vi "Get Property Node Reference.vi"(8 "error in (no error)":errorcluster) -> (0 "error out":errorcluster, 2 "Secondary Prop Refnum":refnum<vi>, 3 "Main Prop Refnum":refnum<vi>)   [LabVIEW 2023]
doc: "<b> </b> <b> </b>\n© 2017 Q Software Innovations, LLC\nwritten by Quentin \"Q\" Alldredge\nproduced in LabVIEW 2015\n\nsupport@qsoftwareinnovations.com\nwww.qsoftwareinnovations.com\n\nAll rights reserved.\n\nRedistribution and use in source and binary forms, with or without modification, are permitted provided that the following conditions are met:\n\n * Redistributions of source code must retain the above copyright notice, this list of conditions and the following disclaimer.\n * Redistributions in binary form must reproduce the above copyright notice, this list of conditions and the following disclaimer in the documentation and/or other materials provided with the distribution.\n * Neither the name of Q Software Innovations, LLC. nor the names of its contributors may be used to endorse or promote products derived from this software without specific prior written permission.\n\nTHIS SOFTWARE IS PROVIDED BY THE COPYRIGHT HOLDERS AND CONTRIBUTORS \"AS IS\" AND ANY EXPRESS OR IMPLIED WARRANTIES, INCLUDING, BUT NOT LIMITED TO, THE IMPLIED WARRANTIES OF MERCHANTABILITY AND FITNESS FOR A PARTICULAR PURPOSE ARE DISCLAIMED. IN NO EVENT SHALL THE COPYRIGHT OWNER OR CONTRIBUTORS BE LIABLE FOR ANY DIRECT, INDIRECT, INCIDENTAL, SPECIAL, EXEMPLARY, OR CONSEQUENTIAL DAMAGES (INCLUDING, BUT NOT LIMITED TO, PROCUREMENT OF SUBSTITUTE GOODS OR SERVICES; LOSS OF USE, DATA, OR PROFITS; OR BUSINESS INTERRUPTION) HOWEVER CAUSED AND ON ANY THEORY OF LIABILITY, WHETHER IN CONTRACT, STRICT LIABILITY, OR TORT (INCLUDING NEGLIGENCE OR OTHERWISE) ARISING IN ANY WAY OUT OF THE USE OF THIS SOFTWARE, EVEN IF ADVISED OF THE POSSIBILITY OF SUCH DAMAGE."
uses:
  <vilib>/Utility/traverseref.llb/VI Scripting - Traverse.lvlib
panel:
  out "exe time (ms)":u32
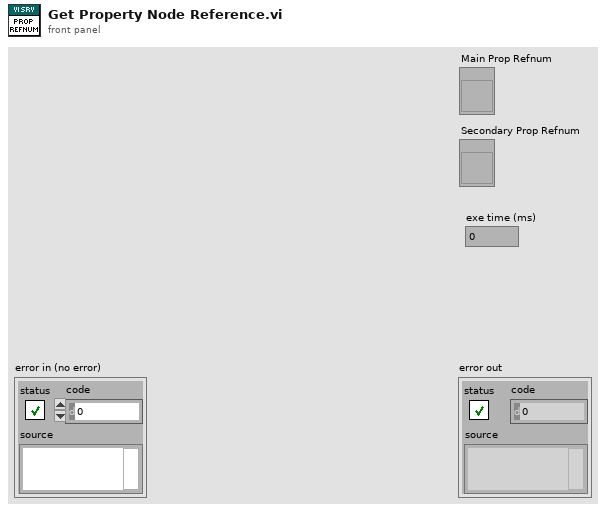
[diagram p1: front panel]
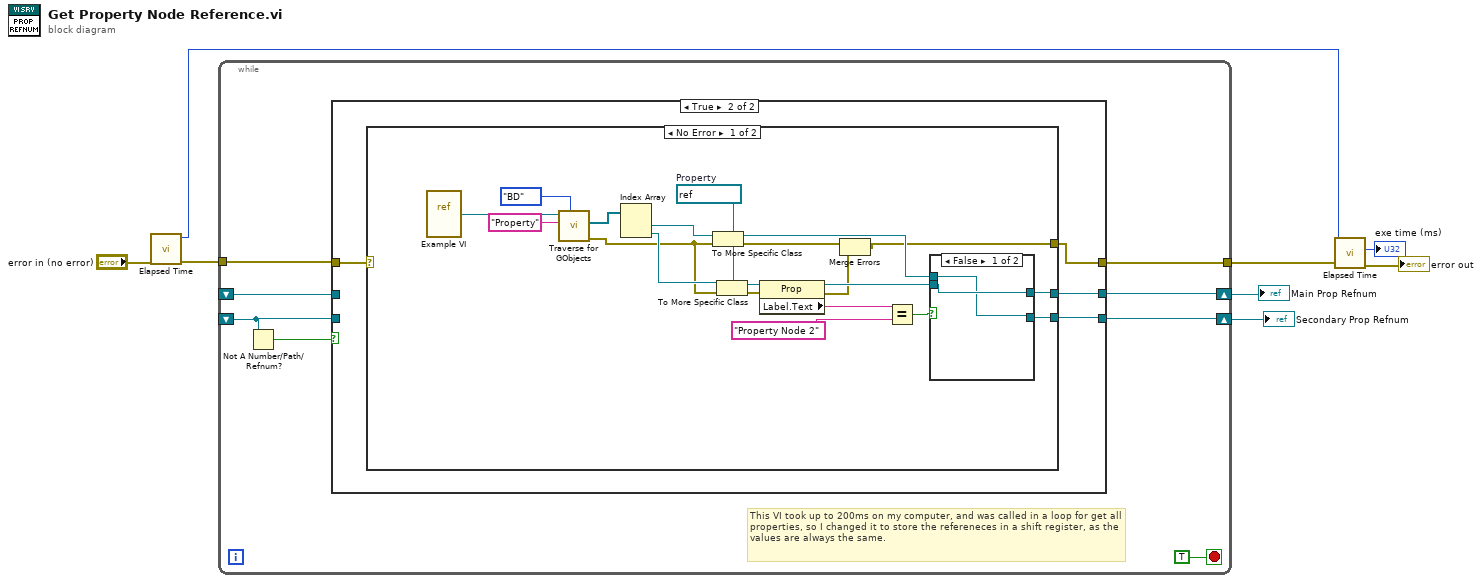
[diagram p0: block diagram]
diagram:
  n1 = call "Elapsed Time.vi"("error in"="error in (no error)") -> ("error out"=w5:errorcluster, "millisecond timer value"=w1:u32)  [unwired: 7 in, 2 out]
  n2 = while {
    shift-right: [w16] -> w8
    shift-left: _ -> [w13]
    shift-right: [w15] -> w7
    shift-left: _ -> [w12]
    tunnel: w5 -> [w11]
    tunnel: [w10] -> w2
    stop <- TRUE stop-if-true
    # "This VI took up to 200ms on my computer, and was called in a loop for get all properties, so I changed it to store the refereneces in a shift register, as the values are always the same."
    n3 = Not A Number/Path/Refnum?(number/path/refnum=w12) -> (NaN/Path/Refnum?=w14:bool)
    n4 = case shown="True" w14 {
      tunnel: w11 -> [w17 w23]
      tunnel: [w19 w22] -> w16
      tunnel: [w18 w21] -> w15
      tunnel: w13 -> [w19 _]
      tunnel: w12 -> [w18 _]
      tunnel: [w17 w20] -> w10
      frame False {
      }
      frame True {
        n5 = case shown="No Error" w23 {
          selector: w23 -> [_ w48]
          tunnel: [w24 w48] -> w20
          tunnel: [w30 _] -> w22
          tunnel: [w32 _] -> w21
          frame No Error {
            w36 = refnum<vi> refnum  # Property
            n6 = vi-ref "Example VI.vi"() -> (w43:refnum<vi>)
            n7 = call <vilib>:"Traverse for GObjects.vi"("Traverse Target"=enum16{"FP", "BD", "Other"}."BD", "Class Name"="Property", "VI Refnum"=w43) -> ("error out"=w27:errorcluster, "References"=w41:refnum<vi>[])  [unwired: 5 in, 2 out]
            n8 = Index Array(array=w41) -> (element #1=w39:refnum<vi>, element #2=w38:refnum<vi>)  [unwired: 2 in]
            n9 = To More Specific Class(target class=w36, reference=w39, error in=w27) -> (specific class reference=w29:refnum<vi>, error out=w28:errorcluster)
            n10 = To More Specific Class(target class=w36, reference=w38, error in=w27) -> (specific class reference=w37:refnum<vi>, error out=w26:errorcluster)
            n11 = property class="Prop"(reference=w37, error in=w26) -> (reference out=w31:refnum<vi>, error out=w25:errorcluster, "Label.Text"=w35:string)
            n12 = Merge Errors(w28, w25) -> (w24:errorcluster)
            n13 = Equal?(x=w35, y="Property Node 2") -> (x = y?=w33:bool)
            n14 = case shown="False" w33 {
              tunnel: [w44 w47] -> w32
              tunnel: w31 -> [w45 w47]
              tunnel: [w45 w46] -> w30
              tunnel: w29 -> [w44 w46]
              frame False {
              }
              frame True {
              }
            }
          }
          frame Error {
          }
        }
      }
    }
  }
  "Main Prop Refnum" <- w8
  "Secondary Prop Refnum" <- w7
  n15 = call "Elapsed Time.vi"("error in"=w2, "past time"=w1) -> ("error out"=→"error out":errorcluster, "elapsed time (ms)"=→"exe time (ms)":u32)  [unwired: 6 in, 2 out]
